vi "get_image.vi"(8 "error in (no error)":errorcluster, 11 "Handle in":u32) -> (0 "error out":errorcluster, 2 "Data":u16[][](array[numeric]), 3 "Handle out":u32)   [LabVIEW 2015]
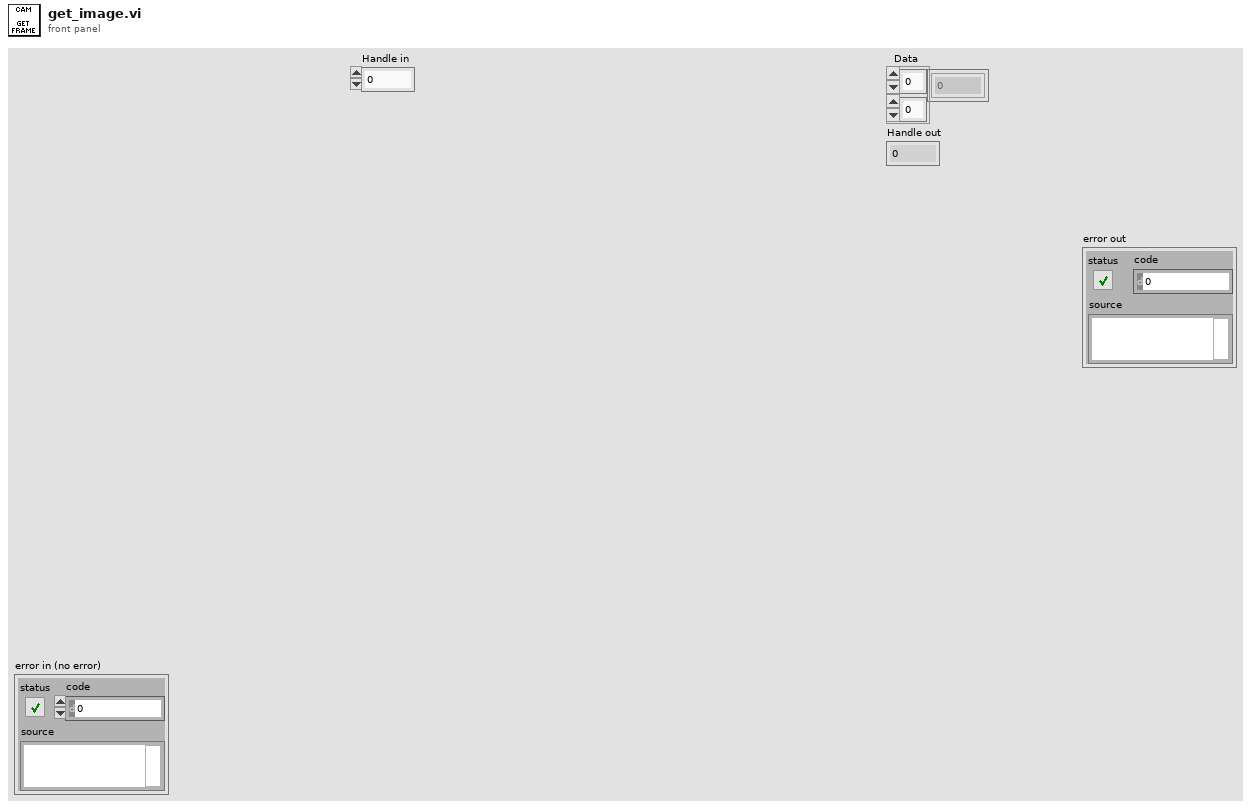
[diagram p1: front panel]
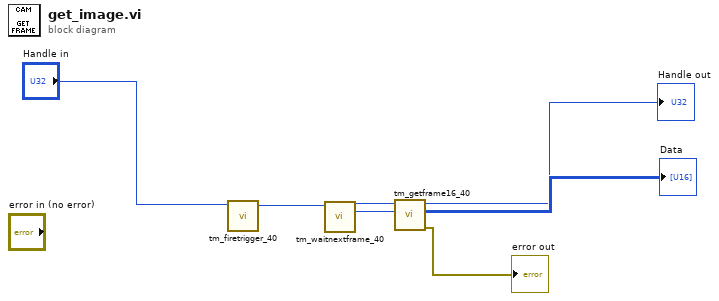
[diagram p0: block diagram]
diagram:
  n1 = call <userlib>:"tm_firetrigger_40.vi"("Handle in"="Handle in") -> ("Handle out"=w7:u32)  [unwired: 9 in, 1 out]
  n2 = call <userlib>:"tm_waitnextframe_40.vi"("Handle in"=w7) -> ("Frame Index"=w5:i32, "Handle out"=w6:u32)  [unwired: 7 in, 2 out]
  n3 = call <userlib>:"tm_getframe16_40.vi"("Frame Index"=w5, "Handle in"=w6) -> ("error out"=→"error out":errorcluster, "Data"=→"Data":u16[][], "Handle out"=→"Handle out":u32)  [unwired: 6 in, 1 out]
